vi "SMO Base Test Launcher (Configurable).vi"() -> ()   [LabVIEW 2013]
uses:
  SMO.lvclass
  Typedefs/SMOState --Enum.ctl
  <vilib>/LabVIEW Open Source/Configuration Manager/Cache/ConfigManager.Cache.lvclass
panel:
  out "error out":errorcluster
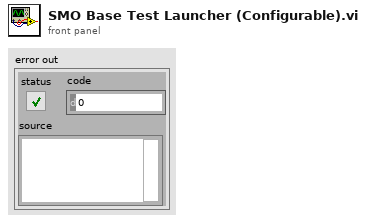
[diagram p1: front panel]
types:
  T1 = typedef "SMO.lvclass/Public Events.ctl" = cluster{"Error":refnum<user-event>, "State":refnum<user-event>, "Reserve State":refnum<user-event>}
  T2 = cluster{"Event Registration Refnum":refnum<event-registration>}
  T3 = typedef "SMO.lvclass/SMOState --Enum.ctl" = enum16{"unknown", "Created", "Started", "Stopped"}
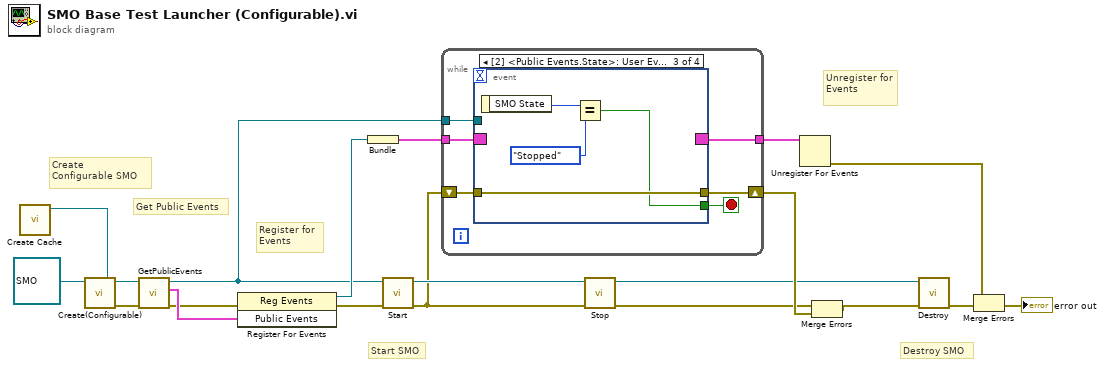
[diagram p0: block diagram]
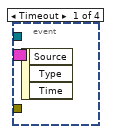
[diagram p2: hidden frame]
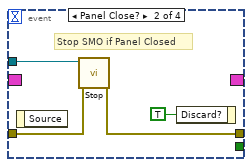
[diagram p3: hidden frame]
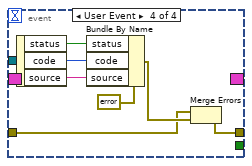
[diagram p4: hidden frame]
diagram:
  # "Get Public Events"
  # "Start SMO"
  # "Destroy SMO"
  # "Create\nConfigurable SMO"
  # "Unregister for Events"
  # "Register for Events"
  n1 = call <vilib>:"Create Cache.vi"() -> ("ConfigManager.Cache"=w1:refnum<class "ConfigManager.Cache.lvclass">)  [unwired: 11 in]
  n2 = call "Create(Configurable).vi"("ConfigManager"=w1, "SMO"=refnum<class "SMO.lvclass"> refnum) -> ("error out"=w2:errorcluster, "SMO out"=w3:refnum<class "SMO.lvclass">)  [unwired: 7 in, 1 out]
  n3 = call "GetPublicEvents.vi"("error in (no error)"=w2, "SMO"=w3) -> ("error out"=w10:errorcluster, "Public Events"=w12:T1, "SMO out"=w11:refnum<class "SMO.lvclass">)  [unwired: 7 in]
  n4 = register-events(error in=w10, w12) -> (reference out=w14:refnum<event-registration>, error out=w13:errorcluster)  [unwired: 1 in]
  n5 = Bundle("Event Registration Refnum"=w14) -> (w19:T2)  [unwired: 1 in]
  n6 = call "Start.vi"("error in (no error)"=w13, "SMO"=w11) -> ("error out"=w6:errorcluster, "SMO out"=w8:refnum<class "SMO.lvclass">)  [unwired: 8 in]
  n7 = while {
    shift-right: [w25] -> w18
    shift-left: w6 -> [w24]
    tunnel: w19 -> [w23]
    tunnel: [w22] -> w20
    tunnel: w11 -> [w21]
    stop <- w26 stop-if-true
    n8 = event shown="[2] <Public Events.State>: User Event" {
      selector: w23 -> [_ _ _ _]
      dyn-events: [_ _ _ _] -> w22
      timeout: _ -> [_ _ _ _]
      tunnel: [_ _ w31 _] -> w26
      tunnel: w21 -> [_ w30 _ _]
      tunnel: [_ w29 w32 w35] -> w25
      tunnel: w24 -> [_ w28 w32 w36]
      event Timeout {
        n9 = event-data() -> ()  [unwired: 1 in, 3 out]
      }
      event Panel Close? {
        # "Stop SMO if Panel Closed"
        n10 = event-data() -> ()  [unwired: 1 in, 1 out]
        n11 = call "Stop.vi"("error in (no error)"=w28, "SMO"=w30) -> ("error out"=w29:errorcluster)  [unwired: 8 in, 1 out]
        n12 = event-data("Discard?"=TRUE ("OK")) -> ()  [unwired: 1 in, 1 out]
      }
      event User Event {
        n13 = event-data() -> ("SMO State"=w34:T3)  [unwired: 1 in]
        n14 = Equal?(x=w34, y=SMOState_--Enum."Stopped") -> (x = y?=w31:bool)
      }
      event User Event {
        n15 = event-data() -> ("status"=w41:bool, "code"=w40:i32, "source"=w39:string)  [unwired: 1 in]
        n16 = Bundle By Name(cluster=errorcluster {"status"=FALSE, "code"=0, "source"=""} ("error out"), "status"=w41, "code"=w40, "source"=w39) -> (w37:errorcluster)
        n17 = Merge Errors(w36, w37) -> (w35:errorcluster)
      }
    }
  }
  n18 = call "Stop.vi"("error in (no error)"=w6, "SMO"=w8) -> ("error out"=w5:errorcluster, "SMO out"=w7:refnum<class "SMO.lvclass">)  [unwired: 8 in]
  n19 = Unregister For Events(event registration refnum=w20) -> (error out=w17:errorcluster)  [unwired: 1 in]
  n20 = Merge Errors(w5, w18) -> (w9:errorcluster)
  n21 = call "Destroy.vi"("error in (no error)"=w9, "SMO"=w7) -> ("error out"=w15:errorcluster)  [unwired: 9 in]
  n22 = Merge Errors(w17, w15) -> (→"error out":errorcluster)
